vi "CP FES GPD and Stim.vi"(8 "Stimulator Controls":T4={"Cluster"={"String 5"="Side", "String"="Stimulator Name", "String 2"="OK", "String 3"="Mode", "String 4"="Timeout (ms)"}, "Left Stimulator Control"={"Side"=enum."Left", "Name"="", "Open"=FALSE, " Mode"="LIVE", "Visa Timeout"=50.0}, "Right Stimulator Control"={"Side"=enum."Right", "Name"="", "Open"=FALSE, " Mode"="LIVE", "Visa Timeout"=50.0}}, 9 "Message from Above":refnum<queue>) -> ()   [LabVIEW 2019]
uses:
  <extravilib>/ChannelInstances/Tag-bool.lvlib
  <extravilib>/ChannelInstances/Event Messenger-bool.lvlib
  Lee Lab/CP FES Walking 2018/Code/Working/LabVIEW/Controls/States/Stim State.ctl
  Lee Lab/CP FES Walking 2018/Code/Working/LabVIEW/Controls/Messages/Stim Message.ctl
  <extravilib>/ChannelInstances/Messenger-t'Stim Message.ctl'.lvlib
  Lee Lab/CP FES Walking 2018/Code/Working/LabVIEW/Controls/States/GPD State.ctl
  Lee Lab/CP FES Walking 2018/Code/Working/LabVIEW/Controls/Messages/GPD Message.ctl
  <extravilib>/ChannelInstances/Messenger-t'GPD Message.ctl'.lvlib
  Lee Lab/CP FES Walking 2018/Code/Working/LabVIEW/Controls/States/Acquisition State.ctl
  Lee Lab/CP FES Walking 2018/Code/Working/LabVIEW/Controls/Messages/Acquisition Message.ctl
  <extravilib>/ChannelInstances/Messenger-t'Acquisition Message.ctl'.lvlib
  Controls/States/CP FES State.ctl
  Controls/Messages/CP FES Message.ctl
  Controls/Left and Right Stim Params.ctl
  Lee Lab/CP FES Walking 2018/Code/Working/LabVIEW/Controls/States/Stim Timer State.ctl
  Lee Lab/CP FES Walking 2018/Code/Working/LabVIEW/Controls/Messages/Stim Timer Message.ctl
  Controls/Protocol Interval.ctl
  Controls/Stim Interval Mode.ctl
  <extravilib>/ChannelInstances/Messenger-t'Stim Timer Message.ctl'.lvlib
  <extravilib>/ChannelInstances/Tag-c(dbl,dbl).lvlib
  <extravilib>/ChannelInstances/Tag-t'Event Data for Plot and Log.ctl'.lvlib
  Controls/Stim off-half-ful.ctl
  Controls/Side Stim Params.ctl
  <extravilib>/ChannelInstances/Messenger-t'Gyro Status Message.ctl'.lvlib
  <extravilib>/ChannelInstances/Messenger-t'Stim Status Message.ctl'.lvlib
  <extravilib>/ChannelInstances/Messenger-t'Timer Status Message.ctl'.lvlib
  Controls/APDM Context Cluster.ctl
  Controls/Stimulator Mode.ctl
  Controls/Type Defs/Stimulator Control_disp.ctl
  Controls/Type Defs/Stimulator Controls.ctl
panel:
  out "Elapsed Time":u32
  in  "input cluster":T3={"Subject Parameter File"=path "", "Initial Interval"={"Interval Type"=enum."Walk", "Duration"=20.0, " Mode"=enum."Stim", "Alt Period"=0.0}, "Stim Protocol Log File"=path ""}
  in  "Right Stim Params":T7
  in  "Left Stim Params":T7
  out "Waveform Chart 3":waveform(dbl)[](graph)
  out "Waveform Chart 2":waveform(i32)[](graph)
  out "Stim Protocol Log File":path
  out "Time to Next Interval":dbl caption="Interval Time (s)" format="%.1f"
  out "Interval Parameters":T1={"Interval Type"=enum."Walk", "Duration"=20.0, " Mode"=enum."Stim", "Alt Period"=0.0}
  out "Timer":i32
  out "Acq":i32
  in  "Init Opals":bool
  out "Stim On/Off":bool
  out "elapsed time":u32
  out "Stim Timer State":T9
  in  "Reload from File":bool
  out "Subject Parameters File":path
  out "Acquisition State":T10
  out "Stim State":T11=enum."Idle"
  out "CP FES State":T12=enum."Initialize"
  in  "VISA Timeout Value":u32=200
  out "Acq iteration duration":u32
  in  "Manual Stim":bool
  in  "Done":bool
  # "Add \"all on/all off\""
  # "Add eccentric/concentric (2D PD and current)"
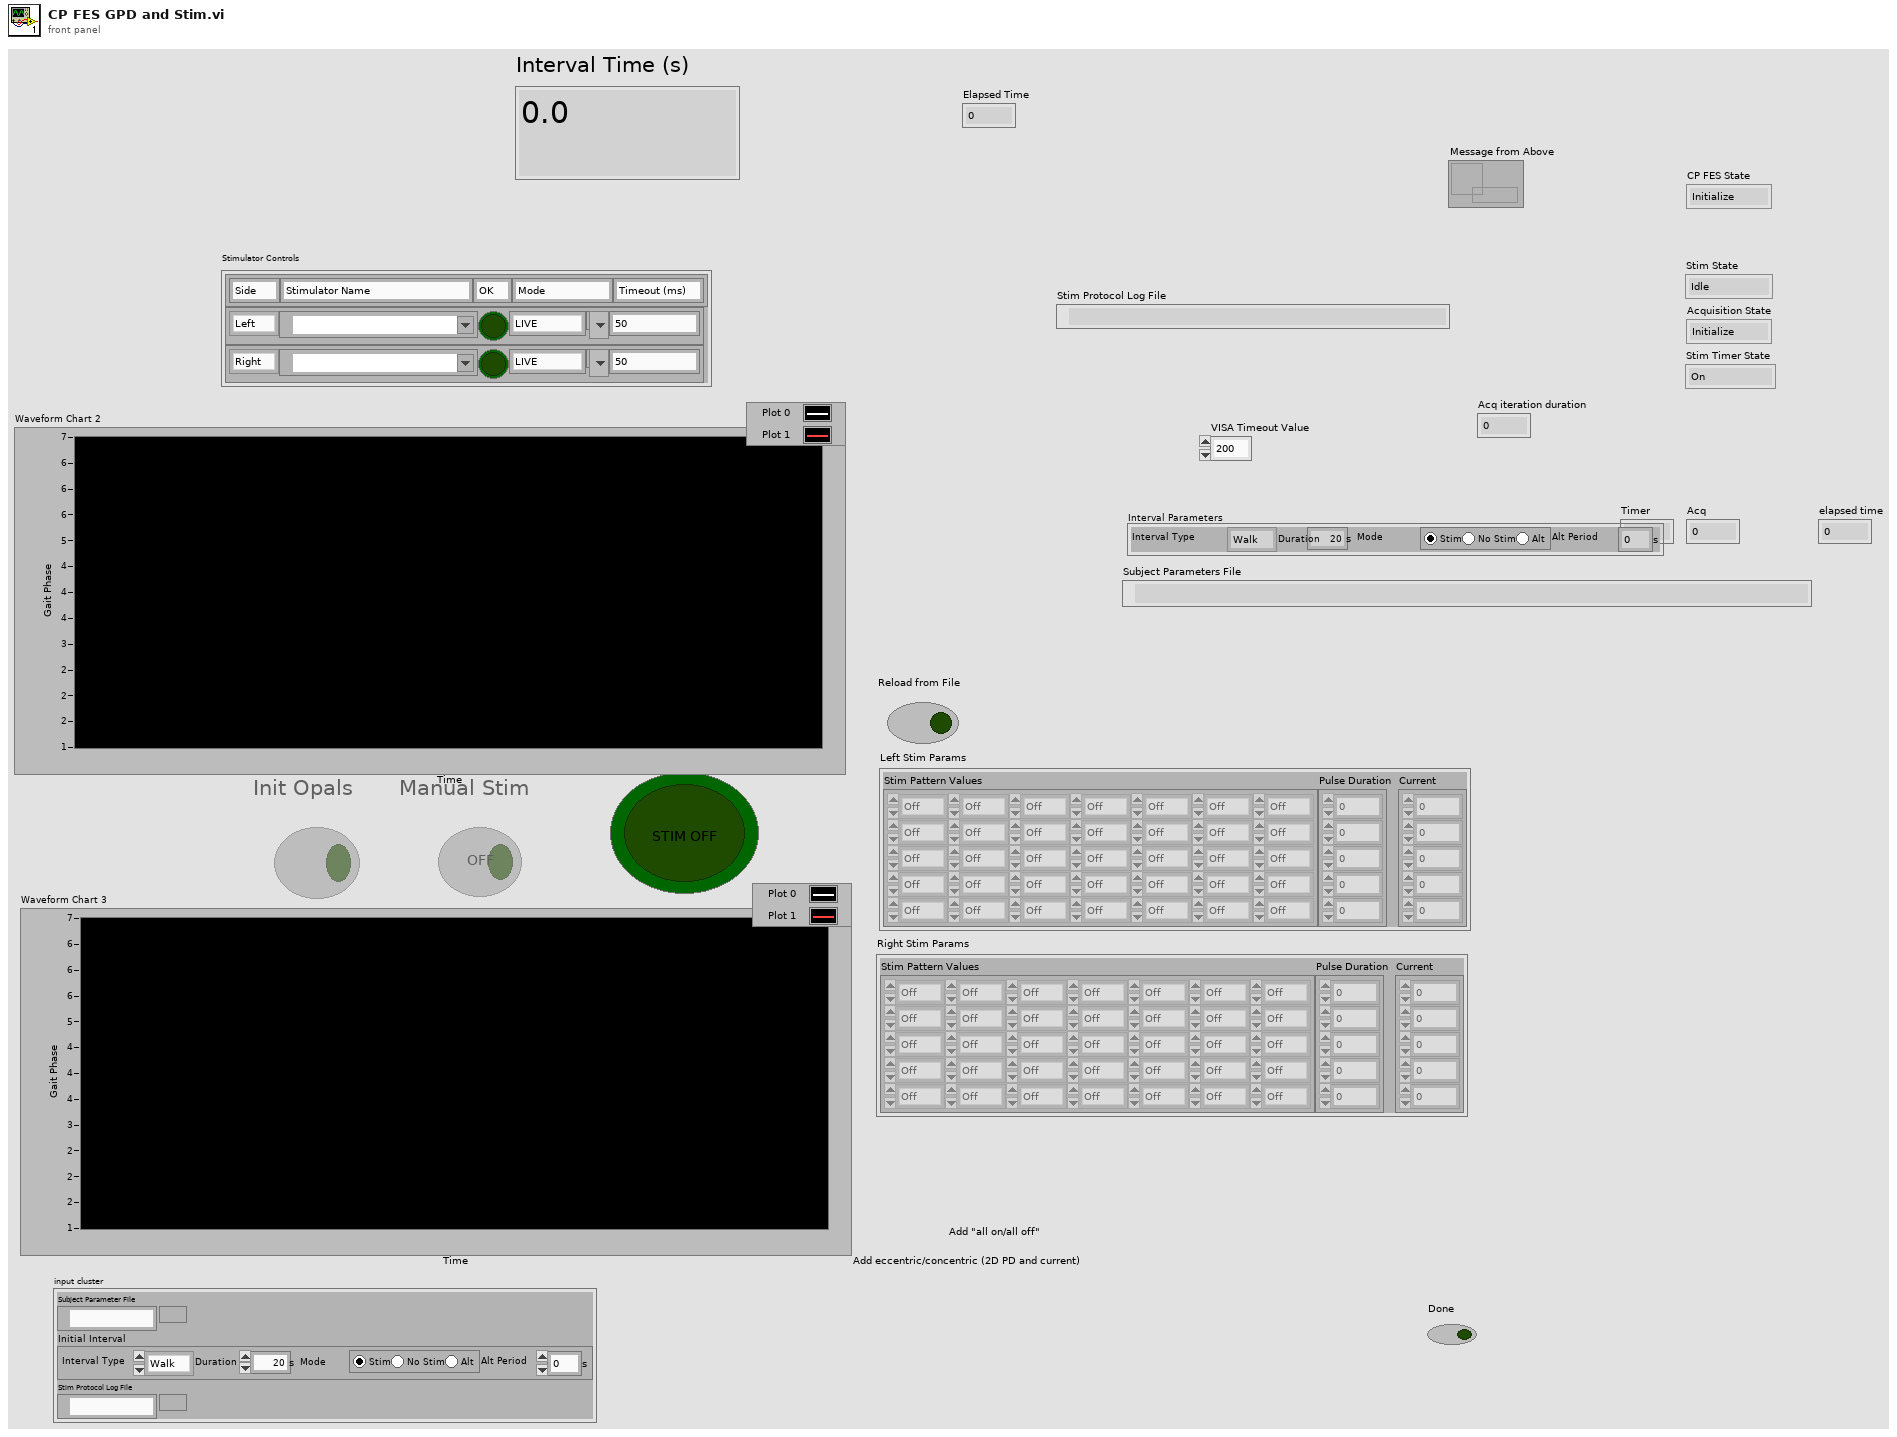
[diagram p1: front panel]
types:
  T1 = typedef "Protocol Interval.ctl" = cluster{"Interval Type":enum16{"Walk", "Rest"}, "Duration":dbl[unit], " Mode":T2, "Alt Period":dbl[unit]}
  T2 = typedef "Stim Interval Mode.ctl" = enum32{"Stim", "No Stim", "Alternating"}
  T3 = cluster{"Subject Parameter File":path, "Initial Interval":T1, "Stim Protocol Log File":path}
  T4 = typedef "Stimulator Controls.ctl" = cluster{"Cluster":cluster{"String 5":string, "String":string, "String 2":string, "String 3":string, "String 4":string}, "Left Stimulator Control":T5, "Right Stimulator Control":T5}
  T5 = typedef "Stimulator Control.ctl" = cluster{"Side":enum16{"Left", "Right"}, "Name":refnum<visa-resource-name>, "Open":bool, " Mode":T6, "Visa Timeout":dbl}
  T6 = typedef "Stimulator Mode.ctl" = string
  T7 = typedef "Side Stim Params.ctl" = cluster{"Stim Pattern Values":T8[][], "Pulse Duration":i64[], "Current":i64[]}
  T8 = typedef "Stim off-half-ful.ctl" = enum16{"Off", "Half", "Full"}
  T9 = typedef "Stim Timer State.ctl" = enum16{"On", "Off", "Initialize", "Stop", "Alternating", "Pause", "Start Timer", "Reset Timer"}
  T10 = typedef "Acquisition State.ctl" = enum16{"Initialize", "Init Hardware", "On", "Off", "Stop"}
  T11 = typedef "Stim State.ctl" = enum16{"Initialize", "Open", "Idle", "Start Stim", "Update Params", "GPD Update", "Stop Stim", "Close", "Quit", "Clear Log"}
  T12 = typedef "CP FES State.ctl" = enum16{"On", "Stop", "Idle", "Initialize", "Manual", "Stim On", "Stim Off", "Start Timer", "Pause", "Resume", "Reset"}
  T13 = typedef "Event Data for Plot and Log.ctl" = cluster{"Event Deteted?":bool, "Event Data":cluster{"Right Event Time":dbl, "Left Event Time":dbl, "Right Phase":i32, "Left Phase":i32}}
  T14 = cluster{"Right Event Time":dbl, "Left Event Time":dbl, "Right Phase":i32, "Left Phase":i32}
  T15 = cluster{"Right Event Time":bool, "Left Event Time":bool, "Right Phase":bool, "Left Phase":bool}
  T16 = cluster{"Right Event Time":dbl, "Left Event Time":dbl, "Right Phase":i32, "Left Phase":i32}[]
  T17 = typedef "CP FES Message.ctl" = cluster{"State":T12, "Data":variant}
  T18 = typedef "Stim Timer Message.ctl" = cluster{"Stim Timer State":T9, "Data":variant}
  T19 = typedef "Stim Message.ctl" = cluster{"Stim State":T11, "Data":variant}
  T20 = typedef "GPD Message.ctl" = cluster{"GPD State":T21, "Data":variant}
  T21 = typedef "GPD State.ctl" = enum16{"On", "Stop", "Idle", "Initialize", "Update GPD Params", "Reload GPD Params", "Detect Event"}
  T22 = typedef "Subject Params.ctl" = cluster{"Subject":T23, "Left GPD Params":T24, "Right GPD Params":T24, "Left Stim Params":T25, "Right Stim Params":T25, "Left Train length":i64[], "Right Train length":i64[]}
  T23 = typedef "Subject.ctl" = u16
  T24 = typedef "GPD Side Parameters.ctl" = cluster{"% Cycle Delay":dbl, "Min % Cycle LR to ISw ":dbl, "Min % Cycle LR to MSw":dbl, "Min % Cycle LR to TSw":dbl, "Max % Cycle ISw to MSw":dbl, "Min % Cycle TSw to LR":dbl, "Max % Cycle TSw to LR":dbl, "LR Min Gyro Z Threshold":dbl, "LR Min Gyro Z Width":dbl, "ISw Peak Threshold":dbl, "ISw Peak Width":dbl, "TSw Valley Threshold":dbl, "TSw Valley Width (ms)":dbl, "Max Cycle Time (s)":dbl, "Mean Computation Window":dbl, "CP subject?":bool}
  T25 = typedef "Stim Parameters.ctl" = cluster{"Stim Pattern Values":T8[][], "Pulse Duration":i64[], "Current":i64[]}
  T26 = typedef "Messenger-t'Stim Timer Message.ctl'.lvlib/))Channel.ctl" = refnum<queue>
  T27 = typedef "Messenger-t'Stim Message.ctl'.lvlib/))Channel.ctl" = refnum<queue>
  T28 = typedef "Messenger-t'GPD Message.ctl'.lvlib/))Channel.ctl" = refnum<queue>
  T29 = typedef "Event Messenger-bool.lvlib/))Channel.ctl" = refnum<queue>
  T30 = enum8{"Enabled", "Disabled", "Disabled and Grayed Out"}
  T31 = typedef "Left and Right Stim Params.ctl" = cluster{"Left Stim Params":T7, "Right Stim Params":cluster{"Stim Pattern Values":T8[][], "Pulse Duration":i64[], "Current":i64[]}}
  T32 = typedef "APDM Context Cluster.ctl" = cluster{"APDM Context ID":u32, "Gyro Mode":string, "Log Data":bool, "Log File":refnum<file>, "Gyro Record Log":refnum<queue>, "Gyro CMD Log":refnum<queue>, "L Opal SN":u32, "R Opal SN":u32, "Access Point ID":u32, "Left Gyro Sim Data":path, "Right Gyro Sim Data":path, "Sampling Rate":dbl, "Gyro Sim Time Array":dbl[], "Missed Gyro Count":dbl}
  T33 = typedef "Acquisition Message.ctl" = cluster{"Acquisition State":T10, "Data":variant}
  T34 = typedef "Messenger-t'Acquisition Message.ctl'.lvlib/))Channel.ctl" = refnum<queue>
  T35 = typedef "Tag-bool.lvlib/))Channel.ctl" = refnum<queue>
  T36 = typedef "Messenger-t'Timer Status Message.ctl'.lvlib/))Channel.ctl" = refnum<queue>
  T37 = typedef "Messenger-t'Gyro Status Message.ctl'.lvlib/))Channel.ctl" = refnum<queue>
  T38 = typedef "Messenger-t'Stim Status Message.ctl'.lvlib/))Channel.ctl" = refnum<queue>
  T39 = typedef "Messenger-t'Log Message.ctl'.lvlib/))Channel.ctl" = refnum<queue>
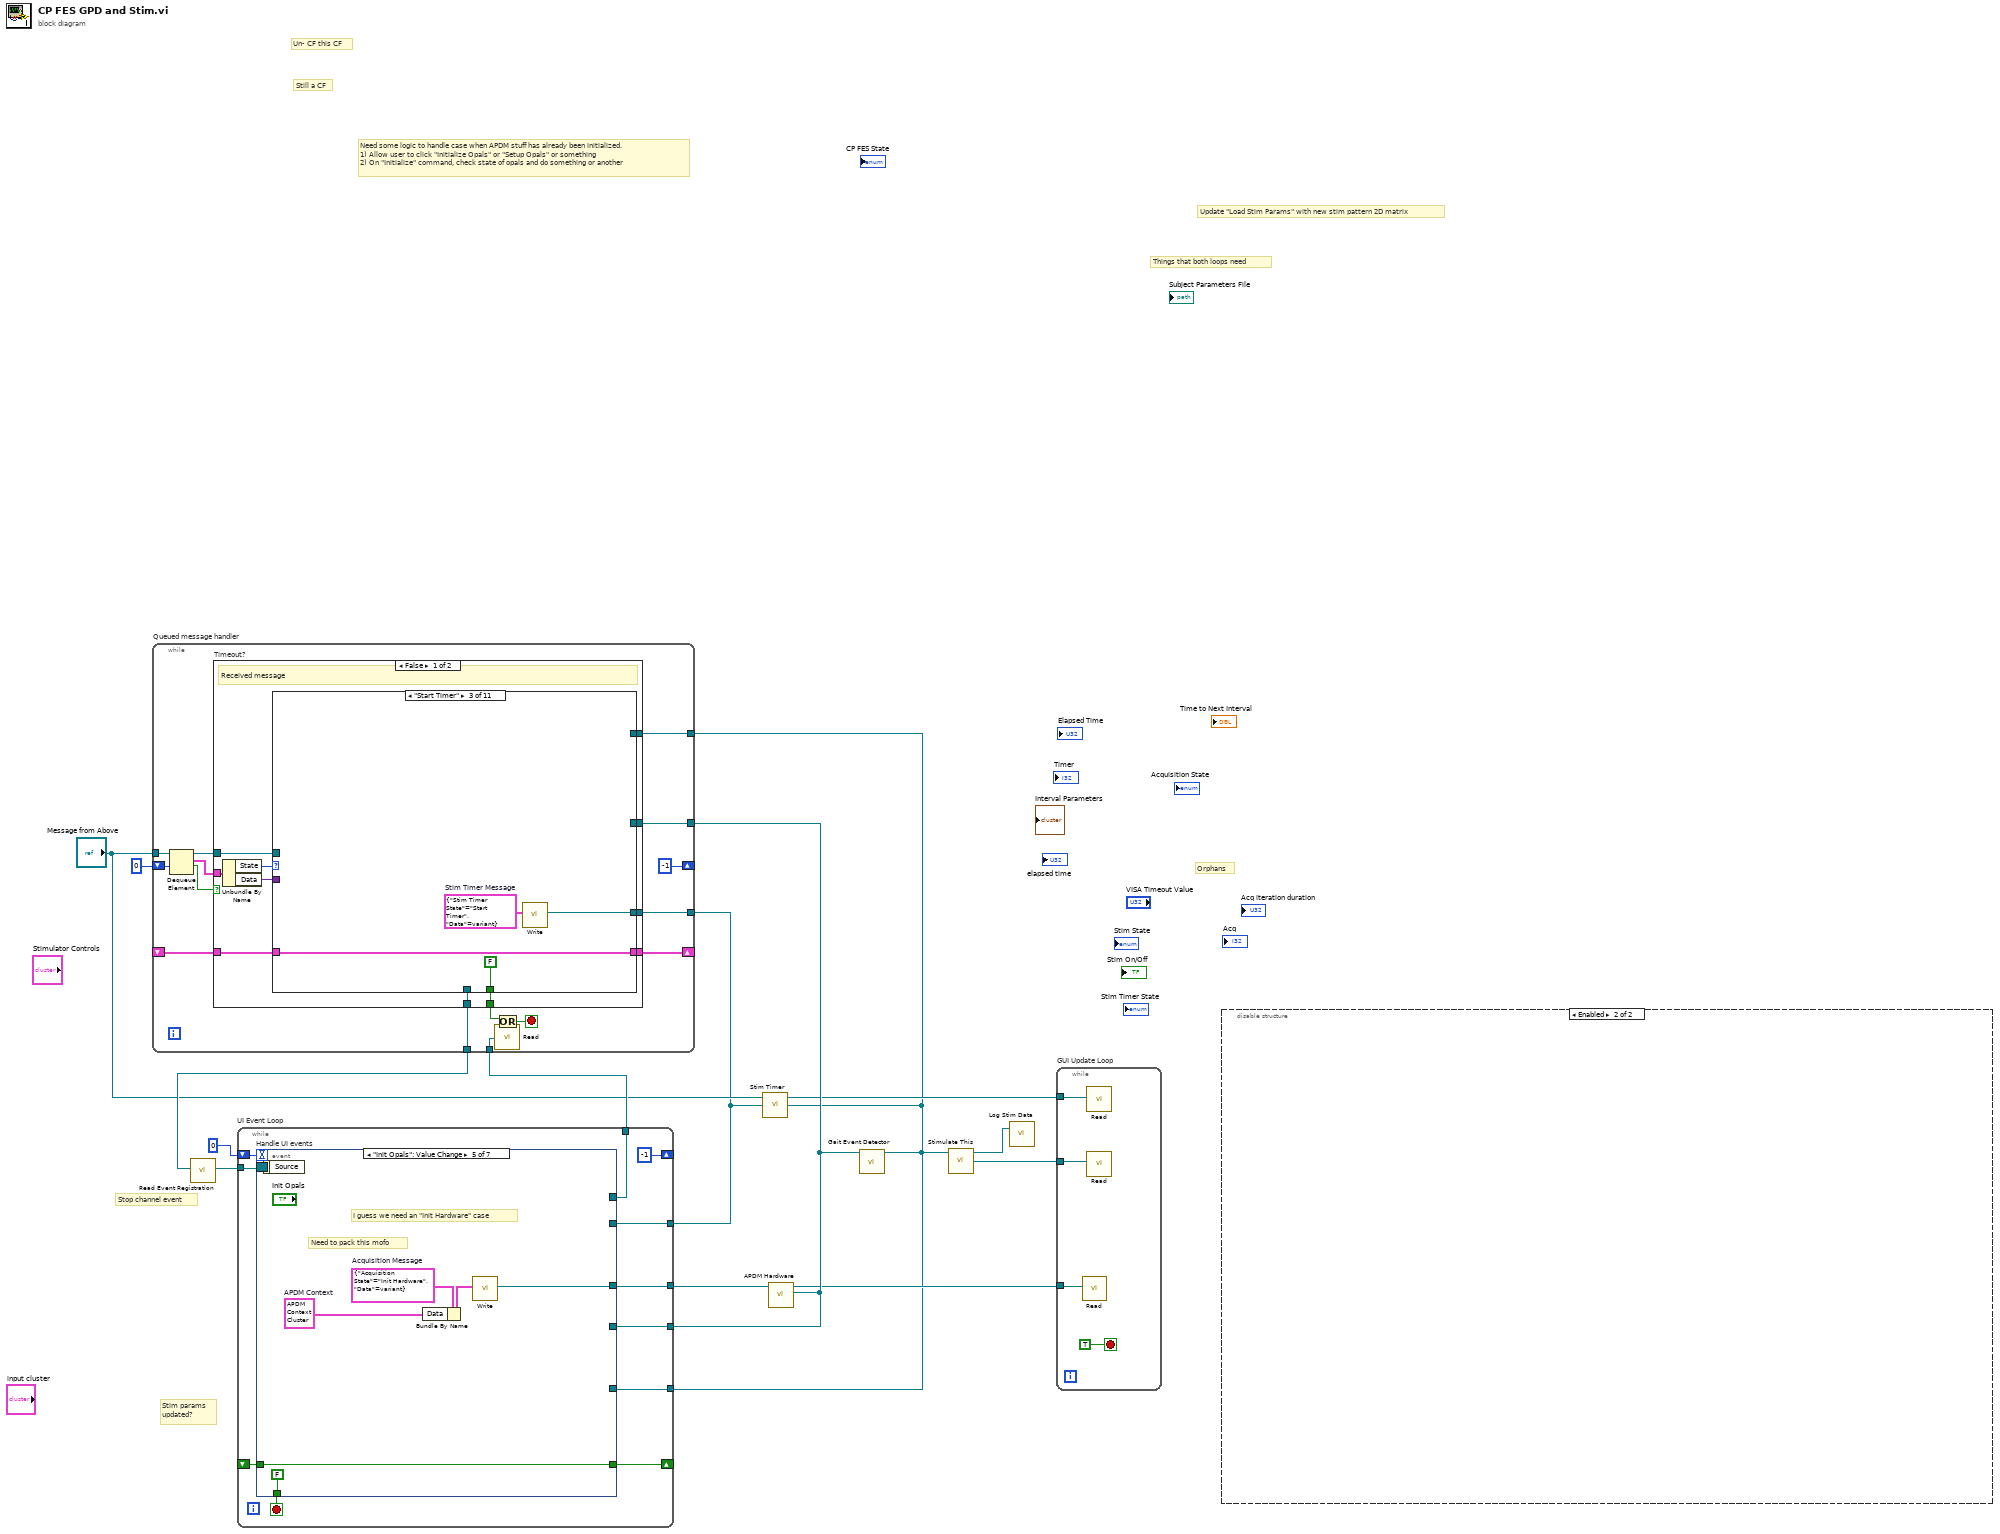
[diagram p0: block diagram]
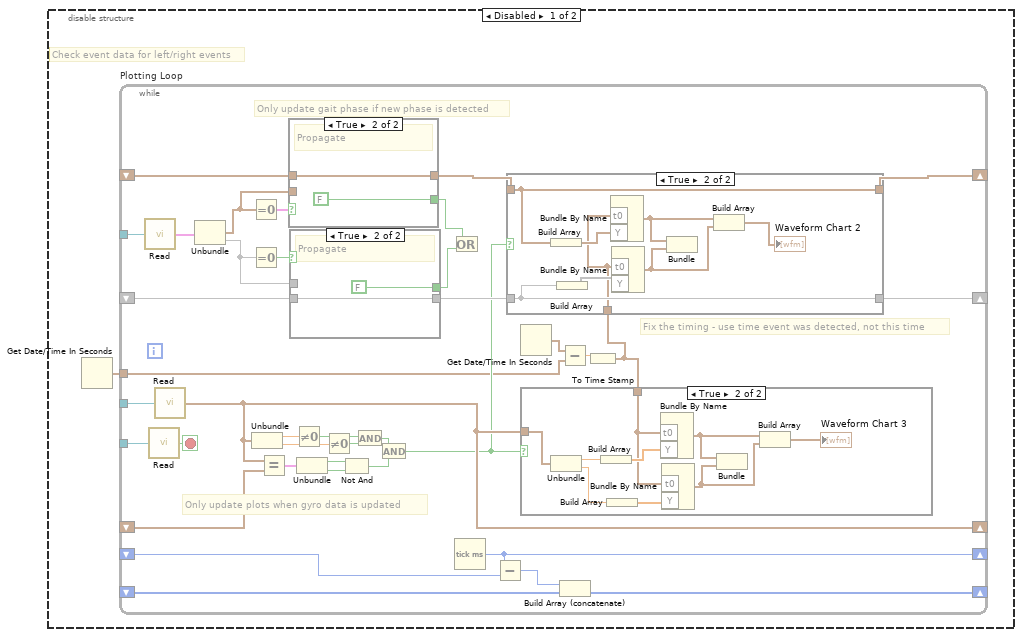
[diagram p2: hidden frame]
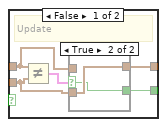
[diagram p5: hidden frame]
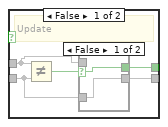
[diagram p7: hidden frame]
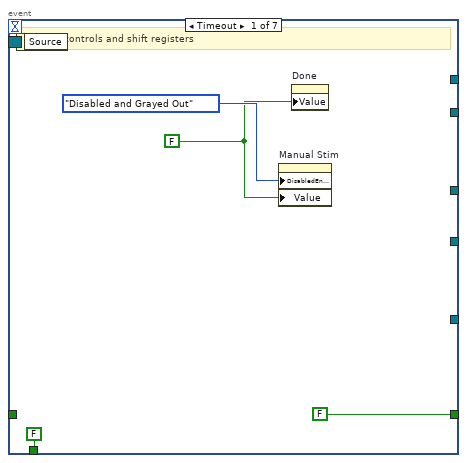
[diagram p9: hidden frame]
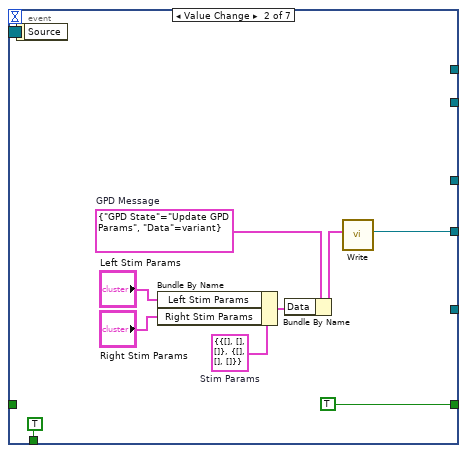
[diagram p10: hidden frame]
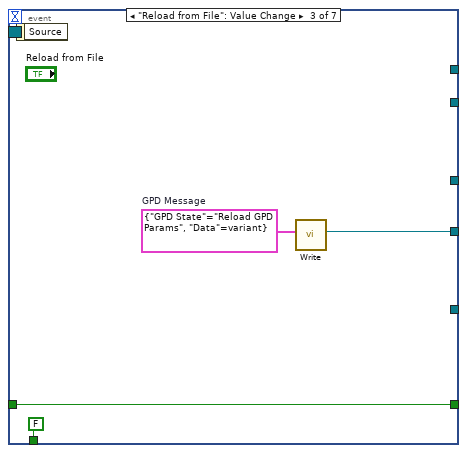
[diagram p11: hidden frame]
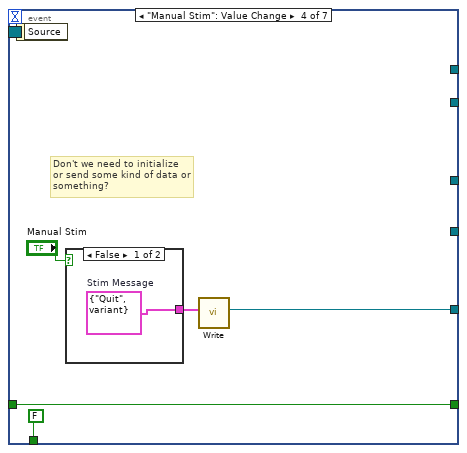
[diagram p12: hidden frame]
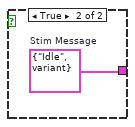
[diagram p13: hidden frame]
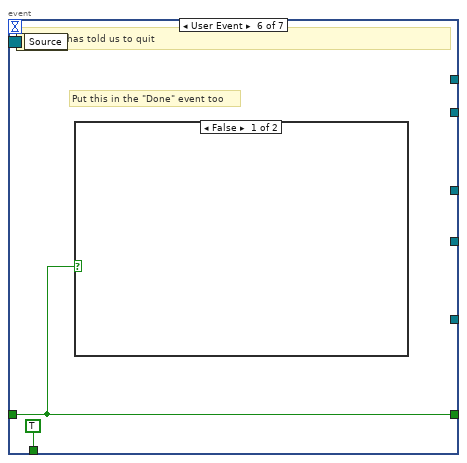
[diagram p14: hidden frame]
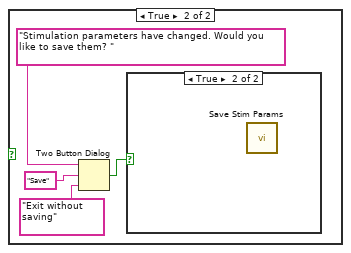
[diagram p15: hidden frame]
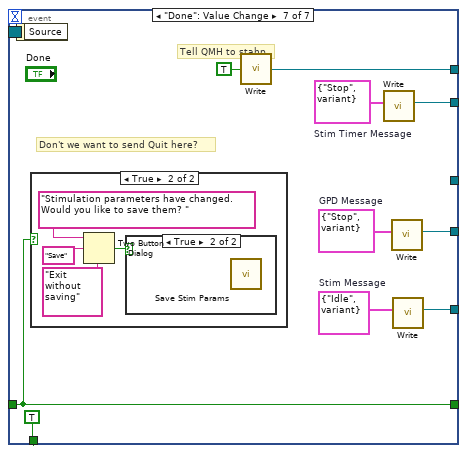
[diagram p17: hidden frame]
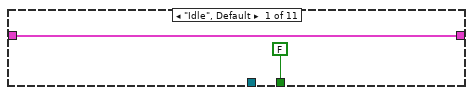
[diagram p20: hidden frame]
diagram:
  # "Stop channel event"
  # "Things that both loops need"
  # "Still a CF"
  # "Un- CF this CF"
  # "Orphans"
  # "Update \"Load Stim Params\" with new stim pattern 2D matrix"
  # "Stim params\nupdated?"
  # "Need some logic to handle case when APDM stuff has already been initialized.\n1) Allow user to click \"Initialize Opals\" or \"Setup Opals\" or something\n2) On \"Initialize\" command, check state of opals and do something or another"
  n1 = disable-structure shown="Enabled" {
    frame Disabled {
      # "Check event data for left/right events"
      n2 = Get Date/Time In Seconds() -> (seconds since 1Jan1904=w18:timestamp)
      n3 = while "Plotting Loop" {
        shift-right: [w48] -> _
        shift-left: _ -> [w47]
        tunnel: [w56] -> w17
        shift-right: [w27] -> _
        shift-left: _ -> [w52]
        shift-right: [w28] -> _
        shift-left: _ -> [w49]
        tunnel: [w40] -> w16
        shift-right: [w37] -> _
        shift-left: _ -> [w36]
        shift-right: [w38] -> _
        shift-left: _ -> [w35]
        tunnel: w18 -> [w24]
        tunnel: [w21] -> w15
        stop <- w39 stop-if-true
        # "Fix the timing - use time event was detected, not this time"
        # "Only update plots when gyro data is updated"
        # "Only update gait phase if new phase is detected"
        n4 = call <extravilib>:"Read.vi"("channel"=w21) -> ("element"=w20:T13)  [unwired: 1 in, 1 out]
        n5 = call <extravilib>:"Read.vi"("channel"=w40) -> ("element"=w39:bool)  [unwired: 1 in, 1 out]
        n6 = call <extravilib>:"Read.vi"("channel"=w56) -> ("element"=w48:cluster{dbl, dbl})  [unwired: 1 in, 1 out]
        n7 = Unbundle(w20) -> (w19:T14, w34)  [unwired: 1 out]
        n8 = Equal To 0?(x=w19) -> (x = 0?=w50:T15)
        n9 = Equal To 0?(x=w34) -> (x = 0?=w51:bool)
        n10 = Unbundle(w48) -> (w46:dbl, w45:dbl)
        n11 = Equal?(x=w48, y=w47) -> (x = y?=w55:cluster{bool, bool})
        n12 = case shown="True" w50 {
          tunnel: [w76 w86] -> w29
          tunnel: w49 -> [w78 w86]
          tunnel: w19 -> [w77 _]
          tunnel: [w80 FALSE ("Boolean")] -> w32
          frame False {
            # "Update"
            n13 = Not Equal?(x=w78, y=w77) -> (x != y?=w79:T15)
            n14 = case shown="True" w79 {
              selector: w79 -> [w81 w83]
              tunnel: [w81 w83] -> w80
              tunnel: w78 -> [w82 _]
              tunnel: w77 -> [_ w84]
              tunnel: [w82 w84] -> w76
              frame False {
              }
              frame True {
              }
            }
          }
          frame True {
            # "Propagate"
          }
        }
        n15 = case shown="True" w51 {
          tunnel: w52 -> [w89 w97]
          tunnel: [w87 w97] -> w30
          tunnel: w34 -> [w88 _]
          tunnel: [w91 FALSE] -> w31
          frame False {
            # "Update"
            n16 = Not Equal?(x=w88, y=w89) -> (x != y?=w90:bool)
            n17 = case shown="False" w90 {
              selector: w90 -> [w93 w95]
              tunnel: [w93 w95] -> w91
              tunnel: w89 -> [w92 _]
              tunnel: w88 -> [_ w94]
              tunnel: [w92 w94] -> w87
              frame False {
              }
              frame True {
              }
            }
          }
          frame True {
            # "Propagate"
          }
        }
        n18 = Not Equal To 0?(x=w46) -> (x != 0?=w44:bool)
        n19 = Unbundle(w55) -> (w54:bool, w53:bool)
        n20 = Not Equal To 0?(x=w45) -> (x != 0?=w43:bool)
        n21 = Not And(1:w53, 2:w54) -> (0:w41:bool)
        n22 = And(x=w44, y=w43) -> (x .and. y?=w42:bool)
        n23 = And(x=w42, y=w41) -> (x .and. y?=w26:bool)
        n24 = Or(x=w32, y=w31) -> ()  [unwired: 1 out]
        n25 = Tick Count (ms)() -> (millisecond timer value=w37:u32)
        n26 = Subtract(x=w37, y=w36) -> (x-y=w33:u32)
        n27 = Get Date/Time In Seconds() -> (seconds since 1Jan1904=w25:timestamp)
        n28 = Subtract(x=w25, y=w24) -> (x-y=w23:dbl)
        n29 = Build Array (concatenate)(w33, w35) -> (w38:u32[])
        n30 = To Time Stamp(1:w23) -> (0:w22:timestamp)
        n31 = case shown="True" w26 {
          tunnel: w30 -> [w57 w63]
          tunnel: w29 -> [w58 w64]
          tunnel: [w58 w64] -> w28
          tunnel: [w57 w63] -> w27
          tunnel: w22 -> [_ w60]
          frame False {
          }
          frame True {
            n32 = Build Array(w64) -> (w66:T16)
            n33 = Build Array(w63) -> (w65:void[])
            n34 = Bundle By Name("t0"=w60, "Y"=w66) -> (w62:waveform(i32))  [unwired: 1 in]
            n35 = Bundle By Name("t0"=w60, "Y"=w65) -> (w61:waveform(i32))  [unwired: 1 in]
            n36 = Bundle(w62, w61) -> ()  [unwired: 1 in, 1 out]
            n37 = Build Array(w62, w61) -> (→"Waveform Chart 2":waveform(i32)[])
          }
        }
        n38 = case shown="True" w26 {
          tunnel: w48 -> [_ w75]
          tunnel: w22 -> [_ w68]
          frame False {
          }
          frame True {
            n39 = Unbundle(w75) -> (w74:dbl, w72:dbl)
            n40 = Build Array(w74) -> (w73:dbl[])
            n41 = Build Array(w72) -> (w71:dbl[])
            n42 = Bundle By Name("t0"=w68, "Y"=w73) -> (w70:waveform(dbl))  [unwired: 1 in]
            n43 = Bundle By Name("t0"=w68, "Y"=w71) -> (w69:waveform(dbl))  [unwired: 1 in]
            n44 = Bundle(w70, w69) -> ()  [unwired: 1 in, 1 out]
            n45 = Build Array(w70, w69) -> (→"Waveform Chart 3":waveform(dbl)[])
          }
        }
      }
    }
    frame Enabled {
    }
  }
  n46 = while "Queued message handler" {
    tunnel: [w113] -> w14
    tunnel: w12 -> [w112]
    tunnel: "Message from Above" -> [w108]
    tunnel: w8 -> [w107]
    tunnel: w3 -> [w106]
    tunnel: w7 -> [w103]
    shift-right: [w102] -> _
    shift-left: _ -> [w101]
    shift-right: [-1] -> _
    shift-left: 0 -> [w99]
    stop <- w109 stop-if-true
    n47 = Dequeue Element(queue=w108, timeout in ms (-1)=w99) -> (queue out=w105:refnum<queue>, element=w104:T17, timed out?=w100:bool)  [unwired: 1 in, 1 out]
    n48 = case "Timeout?" shown="False" w100 {
      tunnel: [w124 _] -> w113
      tunnel: [w123 FALSE] -> w110
      tunnel: [w122 _] -> w107
      tunnel: [w121 _] -> w106
      tunnel: w105 -> [w120 _]
      tunnel: w104 -> [w119 _]
      tunnel: [w118 _] -> w103
      tunnel: [w115 w192] -> w102
      tunnel: w101 -> [w114 w192]
      frame False {
        # "Received message"
        n49 = Unbundle By Name(w119) -> ("State"=w117:T12, "Data"=w116:variant)
        n50 = case shown="\"Start Timer\"" w117 {
          tunnel: [FALSE FALSE FALSE FALSE FALSE FALSE FALSE FALSE FALSE TRUE TRUE] -> w123
          tunnel: [_ _ _ _ _ _ _ _ _ w176 _] -> w124
          tunnel: [_ w144 _ _ _ _ _ _ _ w173 w187] -> w122
          tunnel: [_ w143 _ _ _ _ _ _ _ w172 w185] -> w121
          tunnel: w120 -> [_ w142 _ _ _ _ _ _ _ _ _]
          tunnel: [_ w138 w147 _ _ _ w157 w161 w165 w170 w183] -> w118
          tunnel: [w125 w131 w146 w150 w152 w154 w156 w160 w164 w169 w178] -> w115
          tunnel: w116 -> [_ w130 _ _ _ _ _ _ _ _ w179]
          tunnel: w114 -> [w125 _ w146 w150 w152 w154 w156 w160 w164 w169 w178]
          frame "Idle", Default {
          }
          frame "Initialize" {
            w140 = T18 {"Stim Timer State"=enum."Initialize", "Data"=variant}  # Stim Timer Message
            w141 = T17 {"State"=enum."On", "Data"=variant}  # CP FES Message
            w134 = T19 {"Stim State"=enum."Initialize", "Data"=variant}  # Stim Message
            w133 = T20 {"GPD State"=enum."Initialize", "Data"=variant}  # GPD Message
            # "Make this type def"
            # "Need to add GPD params to this"
            n51 = Variant To Data(type=T3 {"Subject Parameter File"=path "", "Initial Interval"={"Interval Type"=enum."Walk", "Duration"=20.0, " Mode"=enum."Stim", "Alt Period"=0.0}, "Stim Protocol Log File"=path ""} ("input cluster"), Variant=w130) -> (data=w136:T3)  [unwired: 1 in, 1 out]
            n52 = Unbundle By Name(w136) -> ("Stim Protocol Log File"=w127:path, "Initial Interval"=w129:T1, "Subject Parameter File"=w128:path)
            "Stim Protocol Log File" <- w127
            n53 = property on="Time to Next Interval" class="DigNum (strict)"("Visible"=TRUE) -> ()  [unwired: 2 in, 2 out]
            n54 = Enqueue Element(queue=w142, element=w141) -> ()  [unwired: 2 in, 3 out]
            n55 = Bundle By Name(cluster=w140, "Data"=w129) -> (w139:T18)
            n56 = Bundle By Name(cluster=w133, "Data"=w127) -> (w132:T20)
            n57 = call "Load Parameters.vi"("Subject Parameters File"=w128) -> ("Subject Parameters"=w131:T22)  [unwired: 2 in, 2 out]
            n58 = call <extravilib>:"Write.vi"("element"=w139) -> ("channel"=w138:T26)  [unwired: 8 in, 2 out]
            n59 = call <extravilib>:"Write.vi"("element"=w134) -> ("channel"=w143:T27)  [unwired: 8 in, 2 out]
            n60 = call <extravilib>:"Write.vi"("element"=w132) -> ("channel"=w144:T28)  [unwired: 8 in, 2 out]
          }
          frame "Start Timer" {
            w148 = T18 {"Stim Timer State"=enum."Start Timer", "Data"=variant}  # Stim Timer Message
            n61 = call <extravilib>:"Write.vi"("element"=w148) -> ("channel"=w147:T26)  [unwired: 8 in, 2 out]
          }
          frame "On" {
            # "What now?"
          }
          frame "Stim On" {
            # "Prolly need something here"
          }
          frame "Stim Off" {
            # "Here too"
          }
          frame "Pause" {
            w158 = T18 {"Stim Timer State"=enum."Pause", "Data"=variant}  # Stim Timer Message
            n62 = call <extravilib>:"Write.vi"("element"=w158) -> ("channel"=w157:T26)  [unwired: 8 in, 2 out]
          }
          frame "Resume" {
            w162 = T18 {"Stim Timer State"=enum."Start Timer", "Data"=variant}  # Stim Timer Message
            n63 = call <extravilib>:"Write.vi"("element"=w162) -> ("channel"=w161:T26)  [unwired: 8 in, 2 out]
          }
          frame "Reset" {
            w166 = T18 {"Stim Timer State"=enum."Reset Timer", "Data"=variant}  # Stim Timer Message
            n64 = call <extravilib>:"Write.vi"("element"=w166) -> ("channel"=w165:T26)  [unwired: 8 in, 2 out]
          }
          frame "Stop" {
            w171 = T18 {"Stim Timer State"=enum."Stop", "Data"=variant}  # Stim Timer Message
            w174 = T20 {"GPD State"=enum."Stop", "Data"=variant}  # GPD Message
            w175 = T19 {"Stim State"=enum."Idle", "Data"=variant}  # Stim Message
            # "Let stim timer to this too."
            # "Highly questionable (Stim Timer has already stopped stim)"
            # "\"Stop Message\" to event loop"
            n65 = call <extravilib>:"Write.vi"("element"=TRUE) -> ("channel"=w176:T29)  [unwired: 9 in, 1 out]
            n66 = call <extravilib>:"Write.vi"("element"=w175) -> ("channel"=w172:T27)  [unwired: 8 in, 2 out]
            n67 = call <extravilib>:"Write.vi"("element"=w174) -> ("channel"=w173:T28)  [unwired: 8 in, 2 out]
            n68 = call <extravilib>:"Write.vi"("element"=w171) -> ("channel"=w170:T26)  [unwired: 8 in, 2 out]
          }
          frame "Manual" {
            w181 = path ""  # Subject Parameter File
            w184 = T18 {"Stim Timer State"=enum."Off", "Data"=variant}  # Stim Timer Message
            w186 = T19 {"Stim State"=enum."Initialize", "Data"=variant}  # Stim Message
            w188 = T20 {"GPD State"=enum."Initialize", "Data"=variant}  # GPD Message
            w189 = T30."Enabled" ("Disabled")
            # "Wrong VI"
            n69 = Variant To Data(type=w181, Variant=w179) -> (data=w180:path)  [unwired: 1 in, 1 out]
            n70 = property on="Time to Next Interval" class="DigNum (strict)"("Visible"=FALSE) -> ()  [unwired: 2 in, 2 out]
            n71 = call "Load Stim Params.vi"("Stim Parameter Path"=w180) -> ()  [unwired: 3 in, 2 out]
            n72 = property on="Done" class="Bool (strict)"("DisabledEnum"=w189) -> ()  [unwired: 2 in, 2 out]
            n73 = property on="Manual Stim" class="Bool (strict)"("DisabledEnum"=w189) -> ()  [unwired: 2 in, 2 out]
            n74 = call <extravilib>:"Write.vi"("element"=w186) -> ("channel"=w185:T27)  [unwired: 8 in, 2 out]
            n75 = call <extravilib>:"Write.vi"("element"=w188) -> ("channel"=w187:T28)  [unwired: 8 in, 2 out]
            n76 = call <extravilib>:"Write.vi"("element"=w184) -> ("channel"=w183:T26)  [unwired: 8 in, 2 out]
          }
        }
      }
      frame True {
        # "Do initialization stuff"
      }
    }
    n77 = call <extravilib>:"Read.vi"("channel"=w112) -> ("element"=w111:bool)  [unwired: 1 in, 1 out]
    n78 = Or(x=w110, y=w111) -> (x .or. y?=w109:bool)
  }
  n79 = call <extravilib>:"Read Event Registration.vi"("channel"=w14) -> ("event registration refnum"=w13:refnum<event-registration>)  [unwired: 10 in]
  n80 = while "UI Event Loop" {
    tunnel: w13 -> [w202]
    tunnel: [w201] -> w12
    tunnel: [w200] -> w3
    tunnel: [w199] -> w8
    tunnel: [w198] -> w9
    tunnel: [w197] -> w7
    shift-right: [w196] -> _
    shift-left: _ -> [w195]
    shift-right: [-1] -> _
    shift-left: 0 -> [w194]
    stop <- w203 stop-if-true
    n81 = event "Handle UI events" shown="[4] \"Init Opals\": Value Change" {
      selector: w202 -> [_ _ _ _ _ _ _]
      dyn-events: _ -> [_ _ _ _ _ _ _]
      timeout: w194 -> [_ _ _ _ _ _ _]
      tunnel: [FALSE ("Done") TRUE FALSE FALSE FALSE TRUE TRUE ("Done")] -> w203
      tunnel: [_ _ _ _ _ _ w244] -> w201
      tunnel: [_ _ _ w223 _ _ w248] -> w200
      tunnel: [_ w214 w219 _ _ _ w246] -> w199
      tunnel: [_ _ _ _ w233 _ _] -> w198
      tunnel: [_ _ _ _ _ _ w242] -> w197
      tunnel: [FALSE TRUE w217 w221 w231 w234 w240] -> w196
      tunnel: w195 -> [_ _ w217 w221 w231 w234 w240]
      event Timeout {
        w205 = FALSE ("Done")
        # "Initialize controls and shift registers"
        n82 = event-data() -> ()  [unwired: 1 in, 1 out]
        n83 = property on="Manual Stim" class="Bool (strict)"("DisabledEnum"=T30."Disabled and Grayed Out" ("Disabled"), "Value"=w205) -> ()  [unwired: 2 in, 2 out]
        n84 = property on="Done" class="Bool (strict)"("Value"=w205) -> ()  [unwired: 2 in, 2 out]
      }
      event Value Change {
        w211 = T31 {"Left Stim Params"={"Stim Pattern Values"=[], "Pulse Duration"=[], "Current"=[]}, "Right Stim Params"={"Stim Pattern Values"=[], "Pulse Duration"=[], "Current"=[]}}  # Stim Params
        w216 = T20 {"GPD State"=enum."Update GPD Params", "Data"=variant}  # GPD Message
        n85 = event-data() -> ()  [unwired: 1 in, 1 out]
        n86 = Bundle By Name(cluster=w211, "Left Stim Params"="Left Stim Params", "Right Stim Params"="Right Stim Params") -> (w208:T31)
        n87 = Bundle By Name(cluster=w216, "Data"=w208) -> (w215:T20)
        n88 = call <extravilib>:"Write.vi"("element"=w215) -> ("channel"=w214:T28)  [unwired: 8 in, 2 out]
      }
      event "Reload from File": Value Change {
        w220 = T20 {"GPD State"=enum."Reload GPD Params", "Data"=variant}  # GPD Message
        n89 = event-data() -> ()  [unwired: 1 in, 1 out]
        n90 = call <extravilib>:"Write.vi"("element"=w220) -> ("channel"=w219:T28)  [unwired: 8 in, 2 out]
      }
      event "Manual Stim": Value Change {
        # "Don't we need to initialize or send some kind of data or something?"
        n91 = event-data() -> ()  [unwired: 1 in, 1 out]
        n92 = case shown="False" "Manual Stim" {
          tunnel: [w226 w227] -> w224
          frame False {
            w226 = T19 {"Stim State"=enum."Quit", "Data"=variant}  # Stim Message
          }
          frame True {
            w227 = T19 {"Stim State"=enum."Idle", "Data"=variant}  # Stim Message
          }
        }
        n93 = call <extravilib>:"Write.vi"("element"=w224) -> ("channel"=w223:T27)  [unwired: 8 in, 2 out]
      }
      event "Init Opals": Value Change {
        w228 = T32 {"APDM Context ID"=0, "Gyro Mode"="", "Log Data"=FALSE, "Log File"=refnum, "Gyro Record Log"=refnum, "Gyro CMD Log"=refnum, "L Opal SN"=0, "R Opal SN"=0, "Access Point ID"=0, "Left Gyro Sim Data"=path "C:/Users/jfalesi/Desktop/CP FES Walking Code/Original/Ahad Vi/CP Code/Offline data/TD_7_Raw_R.txt", "Right Gyro Sim Data"=path "C:/Users/jfalesi/Desktop/CP FES Walking Code/Original/Ahad Vi/CP Code/Offline data/TD_7_Raw_R.txt", "Sampling Rate"=0.0, "Gyro Sim Time Array"=[], "Missed Gyro Count"=0.0}  # APDM Context
        w230 = T33 {"Acquisition State"=enum."Init Hardware", "Data"=variant}  # Acquisition Message
        # "I guess we need an \"Init Hardware\" case"
        # "Need to pack this mofo"
        n94 = event-data() -> ()  [unwired: 1 in, 1 out]
        n95 = Bundle By Name(cluster=w230, "Data"=w228) -> (w229:T33)
        n96 = call <extravilib>:"Write.vi"("element"=w229) -> ("channel"=w233:T34)  [unwired: 8 in, 2 out]
      }
      event User Event {
        # "Put this in the \"Done\" event too"
        # "Calling VI has told us to quit"
        n97 = event-data() -> ()  [unwired: 1 in, 1 out]
        n98 = case shown="False" w234 {
          frame False {
          }
          frame True {
            n99 = Two Button Dialog(message="Stimulation parameters have changed. Would you like to save them? ", 1:"Exit without saving" ("F button name (\"Cancel\")"), 2:"Save" ("T button name (\"OK\")")) -> (T button?=w236:bool)
            n100 = case shown="True" w236 {
              frame False {
              }
              frame True {
                n101 = call "Save Stim Params.vi"() -> ()  [unwired: 7 in, 1 out]
              }
            }
          }
        }
      }
      event "Done": Value Change {
        w243 = T18 {"Stim Timer State"=enum."Stop", "Data"=variant}  # Stim Timer Message
        w247 = T20 {"GPD State"=enum."Stop", "Data"=variant}  # GPD Message
        w249 = T19 {"Stim State"=enum."Idle", "Data"=variant}  # Stim Message
        # "Tell QMH to stahp"
        # "Don't we want to send Quit here?"
        n102 = event-data() -> ()  [unwired: 1 in, 1 out]
        n103 = case shown="True" w240 {
          frame False {
          }
          frame True {
            n104 = Two Button Dialog(message="Stimulation parameters have changed. Would you like to save them? ", 1:"Exit without saving" ("F button name (\"Cancel\")"), 2:"Save" ("T button name (\"OK\")")) -> (T button?=w250:bool)
            n105 = case shown="True" w250 {
              frame False {
              }
              frame True {
                n106 = call "Save Stim Params.vi"() -> ()  [unwired: 7 in, 1 out]
              }
            }
          }
        }
        n107 = call <extravilib>:"Write.vi"("element"=TRUE) -> ("channel"=w244:T35)  [unwired: 1 out]
        n108 = call <extravilib>:"Write.vi"("element"=w243) -> ("channel"=w242:T26)  [unwired: 8 in, 2 out]
        n109 = call <extravilib>:"Write.vi"("element"=w247) -> ("channel"=w246:T28)  [unwired: 8 in, 2 out]
        n110 = call <extravilib>:"Write.vi"("element"=w249) -> ("channel"=w248:T27)  [unwired: 8 in, 2 out]
      }
    }
  }
  n111 = call "Stim Timer.vi"("Stim Channel"=w3, "Stim Timer Channel"=w7, "Timer Queue"="Message from Above") -> ("Timer Status Channel"=w4:T36)  [unwired: 2 in]
  n112 = call "APDM Hardware.vi"("GPD Message Channel"=w8, "Gyro Channel In"=w9) -> ("Gyro Status Channel"=w6:T37)  [unwired: 5 in]
  n113 = call "Gait Event Detector.vi"("Stim Msg Out"=w3, "GPD Message  In"=w8) -> ()  [unwired: 4 in, 2 out]
  n114 = call "Stimulate This.vi"("Stim Channel"=w3) -> ("Stim Status Channel"=w5:T38, "Stim Log Channel"=w10:T39)  [unwired: 3 in]
  n115 = call "Log Stim Data.vi"("Data Channel"=w10) -> ()  [unwired: 3 in]
  n116 = while "GUI Update Loop" {
    tunnel: w6 -> [w257]
    tunnel: w5 -> [w256]
    tunnel: w4 -> [w255]
    stop <- TRUE stop-if-true
    n117 = call <extravilib>:"Read.vi"("channel"=w257) -> ()  [unwired: 7 in, 4 out]
    n118 = call <extravilib>:"Read.vi"("channel"=w255) -> ()  [unwired: 7 in, 4 out]
    n119 = call <extravilib>:"Read.vi"("channel"=w256) -> ()  [unwired: 7 in, 4 out]
  }
